vi "步进电机初始化.vi"(2 "Z轴速度":dbl, 3 "Y轴速度":dbl, 4 "回零速度":dbl, 5 "细分设置":dbl, 6 "X轴速度":dbl, 7 "串口通信端口":refnum<visa-resource-name>) -> (0 "字符串":string, 1 "串口通信端口O":refnum<visa-resource-name>)   [LabVIEW 2016]
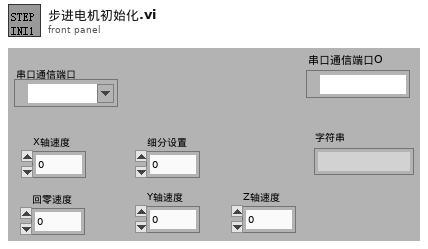
[diagram p1: front panel]
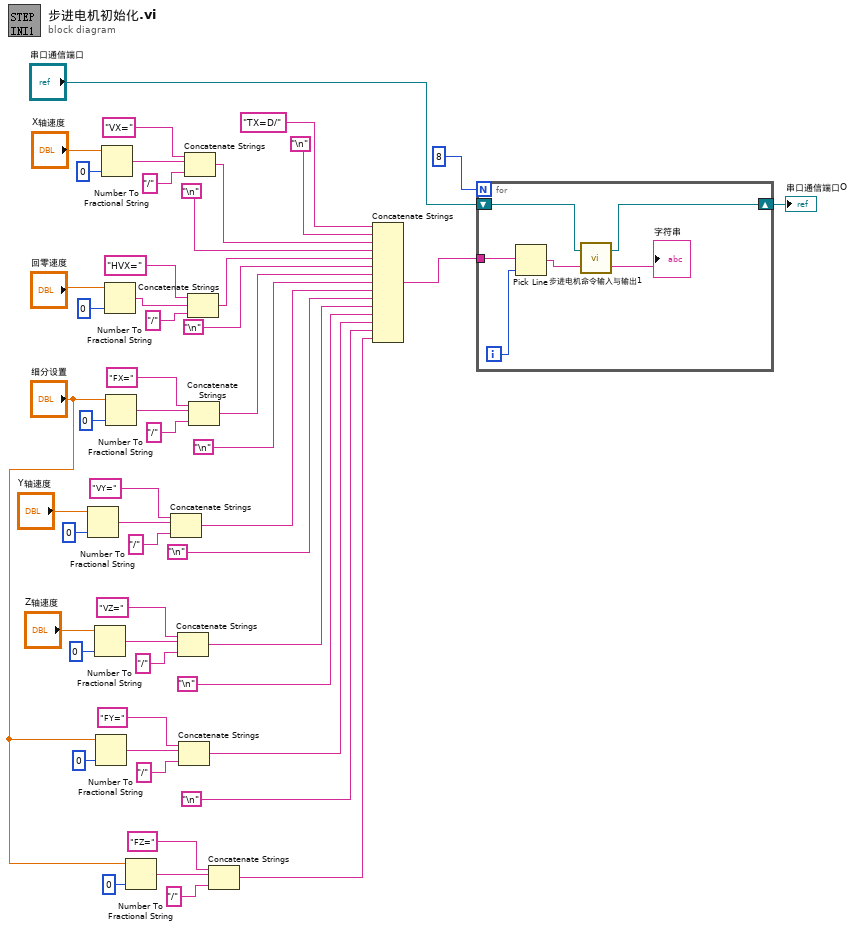
[diagram p0: block diagram]
diagram:
  n1 = Number To Fractional String(number="Y轴速度", precision (6)=i16 0 ("精度(6)")) -> (F-format string=w24:string)  [unwired: 2 out]
  n2 = Number To Fractional String(number="Z轴速度", precision (6)=i16 0 ("精度(6)")) -> (F-format string=w17:string)  [unwired: 2 out]
  n3 = Number To Fractional String(number="细分设置", precision (6)=i16 0 ("精度(6)")) -> (F-format string=w12:string)  [unwired: 2 out]
  n4 = Number To Fractional String(number="X轴速度", precision (6)=i16 0 ("精度(6)")) -> (F-format string=w49:string)  [unwired: 2 out]
  n5 = Number To Fractional String(number="回零速度", precision (6)=i16 0 ("精度(6)")) -> (F-format string=w32:string)  [unwired: 2 out]
  n6 = Number To Fractional String(number="细分设置", precision (6)=i16 0 ("精度(6)")) -> (F-format string=w41:string)  [unwired: 2 out]
  n7 = Number To Fractional String(number="细分设置", precision (6)=i16 0 ("精度(6)")) -> (F-format string=w7:string)  [unwired: 2 out]
  n8 = Concatenate Strings("VY=" ("字符串"), w24, "/" ("字符串")) -> (w22:string)
  n9 = Concatenate Strings("VZ=" ("字符串"), w17, "/" ("字符串")) -> (w15:string)
  n10 = Concatenate Strings("FY=" ("字符串"), w12, "/" ("字符串")) -> (w10:string)
  n11 = Concatenate Strings("VX=" ("字符串"), w49, "/" ("字符串")) -> (w37:string)
  n12 = Concatenate Strings("HVX=" ("字符串"), w32, "/" ("字符串")) -> (w31:string)
  n13 = Concatenate Strings("FX=" ("字符串"), w41, "/" ("字符串")) -> (w29:string)
  n14 = Concatenate Strings("FZ=" ("字符串"), w7, "/" ("字符串")) -> (w4:string)
  n15 = Concatenate Strings("TX=D/" ("字符串"), "\n", w37, "\n", w31, "\n", w29, "\n", w22, "\n", w15, "\n", w10, "\n", w4) -> (w33:string)
  n16 = for {
    N: 8 -> [_]
    tunnel: w33 -> [w56]
    shift-right: [w53] -> w1
    shift-left: "串口通信端口" -> [w58]
    i -> [w57]
    n17 = Pick Line(multi-line string=w56, line index=w57) -> (output string=w55:string)  [unwired: 1 out]
    n18 = call "步进电机命令输入与输出1.vi"("输入字符串"=w55, "串口通信端口"=w58) -> ("返回字符串"=→"字符串":string, "VISA资源名称输出"=w53:refnum<visa-resource-name>)
  }
  "串口通信端口O" <- w1
